vi "Go to Position UM.vi"(7 "V Forward":dbl=3.1, 8 "Goal Frame (World)":cluster{"X":sgl, "Y":sgl, "Theta":dbl}, 9 "Robot Frame (World)":cluster{"X":sgl, "Y":sgl, "Theta":dbl}) -> (2 "Arrive?":bool, 3 "Frame Velocity":dbl[](array[numeric]))   [LabVIEW 2016]
uses:
  <vilib>/Analysis/coordinate.llb/Angle Units.ctl
  <vilib>/Analysis/coordinate.llb/Angle Range (Degree).ctl
  <vilib>/Analysis/coordinate.llb/Wrap Angle (scalar).vi
  <vilib>/Analysis/NI_AAL_Angle.lvlib
panel:
  out "Angle Out (rad)":sgl
  out "coerced(x)":dbl
  out "delta alpha":dbl
  in  "K":dbl=13.0
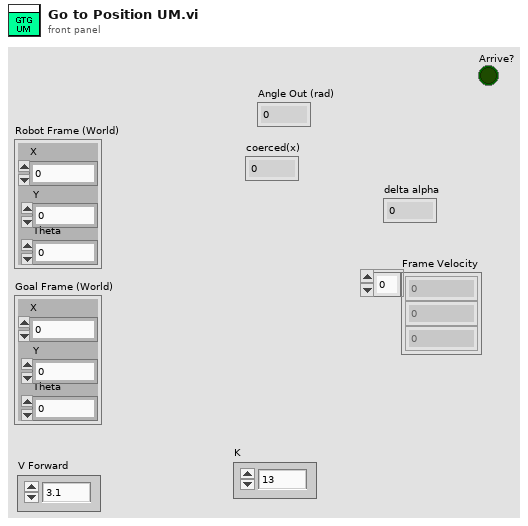
[diagram p1: front panel]
types:
  T1 = typedef "NI_AAL_Angle.lvlib/Angle Range (Degree).ctl" = u16
  T2 = typedef "NI_AAL_Angle.lvlib/Angle Units.ctl" = i32
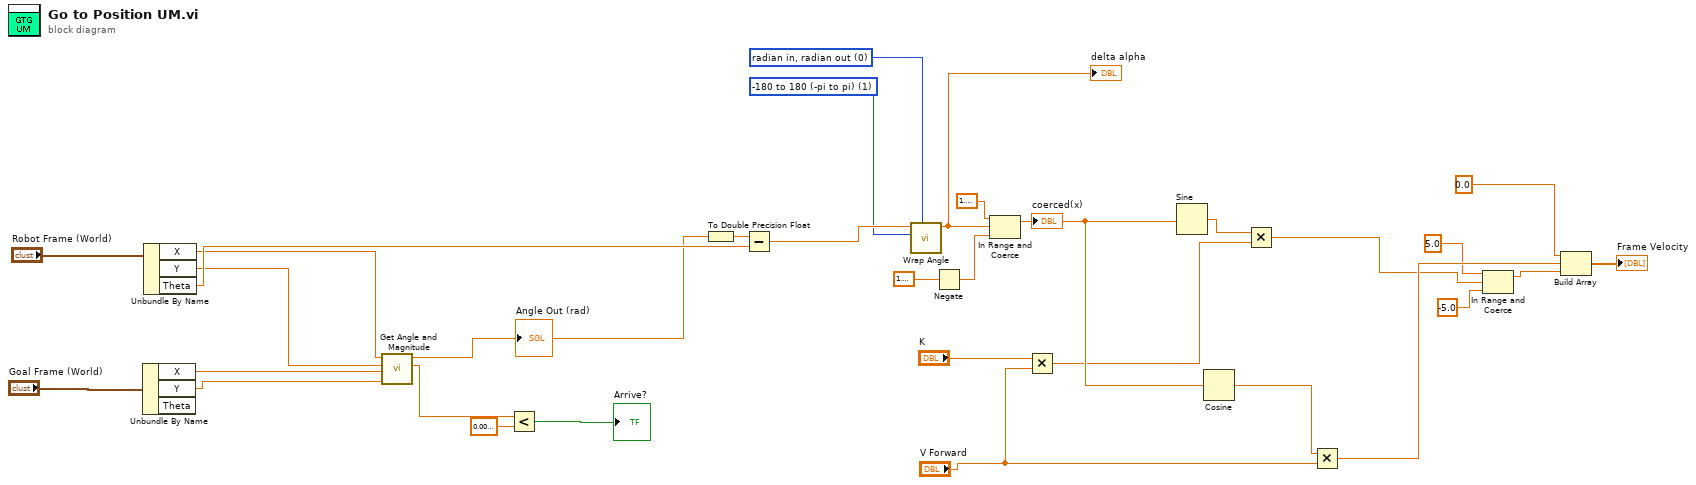
[diagram p0: block diagram]
diagram:
  w28 = T1 1 items=["none", "-180 to 180 (-pi to pi)", "0 to 360 (0 to 2pi)"] ("angle range")
  w29 = T2 0 items=["radian in, radian out", "radian in, degree out", "degree in, degree out", "degree in, radian out"] ("angle units")
  n1 = Unbundle By Name("Goal Frame (World)") -> ("X"=w22:sgl, "Y"=w21:sgl)  [unwired: 1 out]
  n2 = Unbundle By Name("Robot Frame (World)") -> ("X"=w24:sgl, "Y"=w23:sgl, "Theta"=w25:dbl)
  n3 = call "Get Angle and Magnitude.vi"("YGoal"=w21, "XGoal"=w22, "Y"=w23, "X"=w24) -> ("Magnitude"=w7:sgl, "Angle Out (rad)"=w8:sgl)  [unwired: 4 in, 2 out]
  "Angle Out (rad)" <- w8
  n4 = Less?(x=w7, y=sgl 0.01) -> (x < y?=→"Arrive?":bool)
  n5 = To Double Precision Float(number=w8) -> (double precision float=w20:dbl)
  n6 = Subtract(x=w20, y=w25) -> (x-y=w30:dbl)
  n7 = call-poly <vilib>:"Wrap Angle.vi"("angle units"=w29, "angle range"=w28, "angle in"=w30) -> ("angle out"=w18:dbl)  [unwired: 7 in, 1 out]
  "delta alpha" <- w18
  n8 = Negate(x=1.5707963267948966) -> (-x=w15:dbl)
  n9 = In Range and Coerce(upper limit=1.5707963267948966, x=w18, lower limit=w15) -> (coerced(x)=w14:dbl)  [unwired: 1 out]
  "coerced(x)" <- w14
  n10 = Multiply(x="K", y="V Forward") -> (x*y=w10:dbl)
  n11 = Sine(x=w14) -> (sin(x)=w19:dbl)
  n12 = Cosine(x=w14) -> (cos(x)=w13:dbl)
  n13 = Multiply(x=w19, y=w10) -> (x*y=w4:dbl)
  n14 = Multiply(x=w13, y="V Forward") -> (x*y=w12:dbl)
  n15 = In Range and Coerce(upper limit=5.0, x=w4, lower limit=-5.0) -> (coerced(x)=w3:dbl)  [unwired: 1 out]
  n16 = Build Array(0.0 ("index"), w12, w3) -> (→"Frame Velocity":dbl[])
